vi "main.vi"() -> ()   [LabVIEW 2023]
panel:
  out "Flow (sccm)":dbl(slide) scale=0.0..10.0
  out "Power (W)":dbl(knob) scale=0.0..100.0
  out "Ivory OS Input":string
  in  "Control":cluster{"Power":dbl, "Flow":dbl}
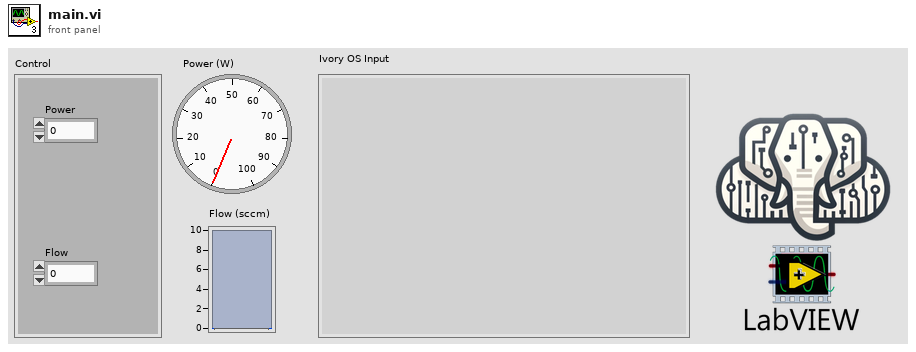
[diagram p1: front panel]
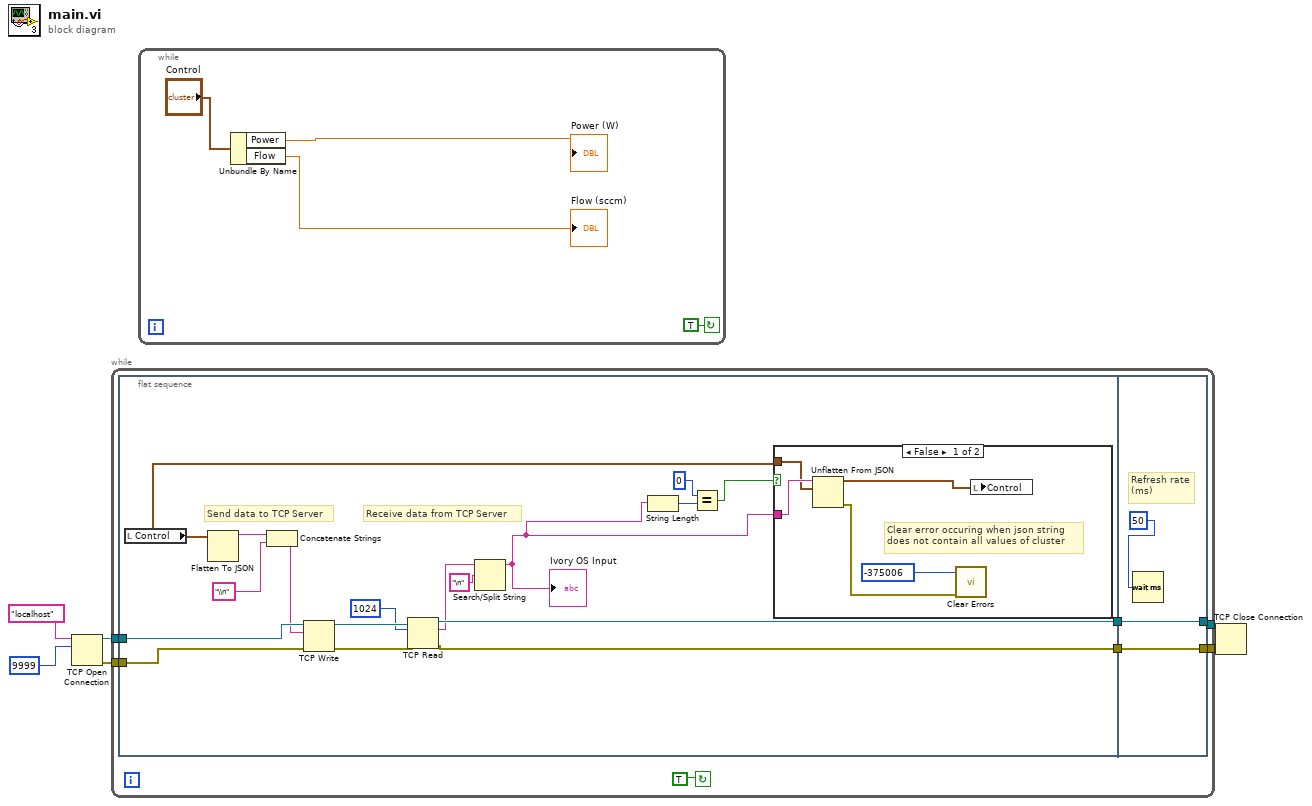
[diagram p0: block diagram]
diagram:
  n1 = TCP Open Connection(address="localhost", remote port or service name=9999) -> (connection ID=w6:refnum<k5>, error out=w5:errorcluster)  [unwired: 3 in]
  n2 = while {
    tunnel: w6 -> [w11]
    tunnel: w5 -> [w12]
    tunnel: [w10] -> w2
    tunnel: [w9] -> w1
    stop <- TRUE continue-if-true
    n3 = flat-sequence {
      tunnel: w12 -> [w30]
      tunnel: w11 -> [w29]
      tunnel: [w27] -> w8
      tunnel: [w25] -> w7
      tunnel: [w37] -> w9
      tunnel: [w38] -> w10
      tunnel: w8 -> [w38]
      tunnel: w7 -> [w37]
      frame #0 {
        # "Receive data from TCP Server"
        # "Send data to TCP Server"
        n4 = local read "Control"() -> (w15:cluster{"Power":dbl, "Flow":dbl})
        n5 = Flatten To JSON(anything=w15) -> (JSON string=w23:string)  [unwired: 2 in, 1 out]
        n6 = Concatenate Strings(w23, "\\n") -> (w22:string)
        n7 = TCP Write(connection ID=w29, data in=w22, error in (no error)=w30) -> (connection ID out=w26:refnum<k5>, error out=w28:errorcluster)  [unwired: 1 in, 1 out]
        n8 = TCP Read(connection ID=w26, bytes to read=1024, error in (no error)=w28) -> (connection ID out=w25:refnum<k5>, data out=w20:string, error out=w27:errorcluster)  [unwired: 2 in]
        n9 = Search/Split String(string=w20, search string/char (-)="\n") -> (substring before match=w16:string)  [unwired: 1 in, 2 out]
        "Ivory OS Input" <- w16
        n10 = String Length(string=w16) -> (length=w18:i32)
        n11 = Equal?(x=0, y=w18) -> (x = y?=w14:bool)
        n12 = case shown="False" w14 {
          tunnel: w16 -> [w35 _]
          tunnel: w15 -> [w34 _]
          frame False {
            # "Clear error occuring when json string\ndoes not contain all values of cluster"
            n13 = Unflatten From JSON(JSON string=w35, type and defaults=w34) -> (value=w33:cluster{"Power":dbl, "Flow":dbl}, error out=w32:errorcluster)  [unwired: 5 in]
            n14 = call <vilib>:"Clear Errors.vi"("error in (no error)"=w32, "specific error code to clear (0: all)"=-375006) -> ()  [unwired: 4 in, 2 out]
            n15 = local write "Control"(w33) -> ()
          }
          frame True {
          }
        }
      }
      frame #1 {
        # "Refresh rate\n(ms)"
        n16 = Wait (ms)(milliseconds to wait=50) -> ()  [unwired: 1 out]
      }
    }
  }
  n17 = while {
    stop <- TRUE continue-if-true
    n18 = Unbundle By Name("Control") -> ("Power"=→"Power (W)":dbl, "Flow"=→"Flow (sccm)":dbl)
  }
  n19 = TCP Close Connection(connection ID=w1, error in (no error)=w2) -> ()  [unwired: 1 in, 2 out]
